vi "Keithley 6430 Bias.vi"() -> ()   [LabVIEW 2014]
uses:
  Environmental Chamber LabVIEW and Instruments/Drivers and Software/keithley_6430/Keithley 6430/Keithley 6430.lvlib
panel:
  in  "Bias (V)":dbl min=-190.0 max=190.0
  in  "Stop Button":bool
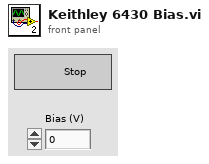
[diagram p1: front panel]
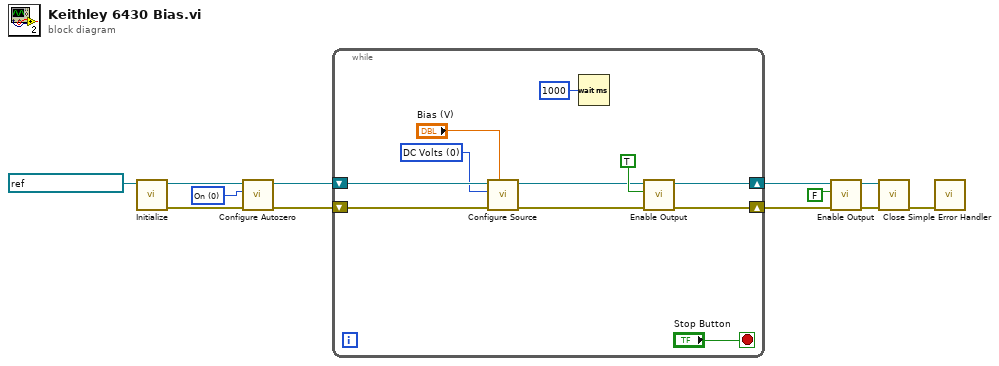
[diagram p0: block diagram]
diagram:
  w9 = u16 0 items=["On", "Off", "Once"] ("Autozero  (0: On)")
  n1 = call "Initialize.vi"("VISA resource name"=refnum<visa-resource-name> "GPIB2::19::INSTR") -> ("error out"=w10:errorcluster, "VISA resource name out"=w11:refnum<visa-resource-name>)  [unwired: 4 in, 5 out]
  n2 = call "Configure Autozero.vi"("error in (no error)"=w10, "Autozero  (0: On)"=w9, "VISA resource name"=w11) -> ("error out"=w7:errorcluster, "VISA resource name out"=w8:refnum<visa-resource-name>)  [unwired: 7 in]
  n3 = while {
    shift-right: [w19] -> w2
    shift-left: w8 -> [w22]
    shift-right: [w18] -> w1
    shift-left: w7 -> [w21]
    stop <- "Stop Button" stop-if-true
    w20 = u16 0 items=["DC Volts", "DC Current"] ("Source Function (0: DC Volts)")
    n4 = call "Configure Source.vi"("V-Source Level [V]"="Bias (V)", "error in (no error)"=w21, "Source Function (0: DC Volts)"=w20, "VISA resource name"=w22) -> ("error out"=w13:errorcluster, "VISA resource name out"=w14:refnum<visa-resource-name>)  [unwired: 6 in]
    n5 = Wait (ms)(milliseconds to wait=u32 1000) -> ()  [unwired: 1 out]
    n6 = call "Enable Output.vi"("error in (no error)"=w13, "Enable Output (F:Off)"=TRUE ("Output (F:Off)"), "VISA resource name"=w14) -> ("error out"=w18:errorcluster, "VISA resource name out"=w19:refnum<visa-resource-name>)  [unwired: 7 out]
  }
  n7 = call "Enable Output.vi"("error in (no error)"=w1, "Enable Output (F:Off)"=FALSE ("Output (F:Off)"), "VISA resource name"=w2) -> ("error out"=w4:errorcluster, "VISA resource name out"=w5:refnum<visa-resource-name>)  [unwired: 7 out]
  n8 = call "Close.vi"("error in (no error)"=w4, "VISA resource name"=w5) -> ("error out"=w3:errorcluster)  [unwired: 9 out]
  n9 = call <vilib>:"Simple Error Handler.vi"("error in (no error)"=w3) -> ()  [unwired: 4 in, 5 out]
